vi "RichToFlatGreeter_req.vi"(5 "OutputClusterType":T1, 11 "InputCluster":T2) -> (3 "OutputCluster":T1)   [LabVIEW 2019, in "Generated_server.lvlib"]
uses:
  Generated_server.lvlib
  Greeter_req.ctl
  Greeter_req_req_oneof/Greeter_req_req_oneof.lvclass
  Greeter_req_Flat.ctl
  Greeter_req_req_oneof/Greeter_req_req_oneof.lvclass/Greeter_req_req_oneof.ctl
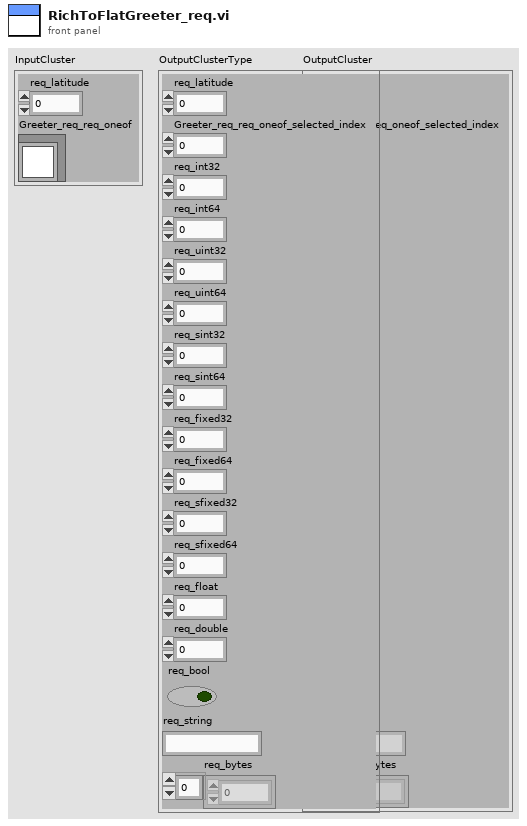
[diagram p1: front panel]
types:
  T1 = typedef "Generated_server.lvlib/Greeter_req_Flat.ctl" = cluster{"req_latitude":i32, "Greeter_req_req_oneof_selected_index":i32, "req_int32":i32, "req_int64":i64, "req_uint32":u32, "req_uint64":u64, "req_sint32":i32, "req_sint64":i64, "req_fixed32":u32, "req_fixed64":u64, "req_sfixed32":i32, "req_sfixed64":i64, "req_float":sgl, "req_double":dbl, "req_bool":bool, "req_string":string, "req_bytes":u8[]}
  T2 = typedef "Generated_server.lvlib/Greeter_req.ctl" = cluster{"req_latitude":i32, "Greeter_req_req_oneof":refnum<class "Greeter_req_req_oneof.lvclass">}
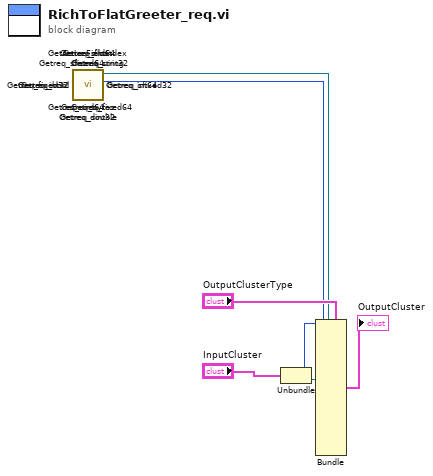
[diagram p0: block diagram]
diagram:
  n1 = Unbundle "Unbundle"("InputCluster") -> ("req_latitude"=w18:i32, "Greeter_req_req_oneof"=w17:refnum<class "Greeter_req_req_oneof.lvclass">)
  n2 = call "Getreq_bytes.vi"("OneOfTemplate in"=w17) -> ("Get_Val"=w1:u8[])  [unwired: 8 in, 2 out]
  n3 = call "Getreq_string.vi"("OneOfTemplate in"=w17) -> ("Get_Val"=w2:string)  [unwired: 8 in, 2 out]
  n4 = call "Getreq_bool.vi"("OneOfTemplate in"=w17) -> ("Get_Val"=w3:bool)  [unwired: 8 in, 2 out]
  n5 = call "Getreq_double.vi"("OneOfTemplate in"=w17) -> ("Get_Val"=w4:dbl)  [unwired: 8 in, 2 out]
  n6 = call "Getreq_float.vi"("OneOfTemplate in"=w17) -> ("Get_Val"=w5:sgl)  [unwired: 8 in, 2 out]
  n7 = call "Getreq_sfixed64.vi"("OneOfTemplate in"=w17) -> ("Get_Val"=w6:i64)  [unwired: 8 in, 2 out]
  n8 = call "Getreq_sfixed32.vi"("OneOfTemplate in"=w17) -> ("Get_Val"=w7:i32)  [unwired: 8 in, 2 out]
  n9 = call "Getreq_fixed64.vi"("OneOfTemplate in"=w17) -> ("Get_Val"=w8:u64)  [unwired: 8 in, 2 out]
  n10 = call "Getreq_fixed32.vi"("OneOfTemplate in"=w17) -> ("Get_Val"=w9:u32)  [unwired: 8 in, 2 out]
  n11 = call "Getreq_sint64.vi"("OneOfTemplate in"=w17) -> ("Get_Val"=w10:i64)  [unwired: 8 in, 2 out]
  n12 = call "Getreq_sint32.vi"("OneOfTemplate in"=w17) -> ("Get_Val"=w11:i32)  [unwired: 8 in, 2 out]
  n13 = call "Getreq_uint64.vi"("OneOfTemplate in"=w17) -> ("Get_Val"=w12:u64)  [unwired: 8 in, 2 out]
  n14 = call "Getreq_uint32.vi"("OneOfTemplate in"=w17) -> ("Get_Val"=w13:u32)  [unwired: 8 in, 2 out]
  n15 = call "Getreq_int64.vi"("OneOfTemplate in"=w17) -> ("Get_Val"=w14:i64)  [unwired: 8 in, 2 out]
  n16 = call "Getreq_int32.vi"("OneOfTemplate in"=w17) -> ("Get_Val"=w15:i32)  [unwired: 8 in, 2 out]
  n17 = call "GetActiveFieldIndex.vi"("OneOfTemplate in"=w17) -> ("Active Field Index"=w16:i32)  [unwired: 8 in, 2 out]
  n18 = Bundle "Bundle"(cluster="OutputClusterType", "req_latitude"=w18, "Greeter_req_req_oneof_selected_index"=w16, "req_int32"=w15, "req_int64"=w14, "req_uint32"=w13, "req_uint64"=w12, "req_sint32"=w11, "req_sint64"=w10, "req_fixed32"=w9, "req_fixed64"=w8, "req_sfixed32"=w7, "req_sfixed64"=w6, "req_float"=w5, "req_double"=w4, "req_bool"=w3, "req_string"=w2, "req_bytes"=w1) -> (→"OutputCluster":T1)
